vi "Frame to Data.vi"(10 "Frame":string) -> (0 "element":string[](array[string]), 1 "MulFrame":bool, 2 "Array":u8[](array[numeric]), 3 "Get Key？":bool, 4 "Finish":bool, 5 "Error？":bool)   [LabVIEW 2018]
uses:
  <vilib>/regexp/Match Regular Expression.xnode
panel:
  out "Numeric":i32
  out "offset past match":i32
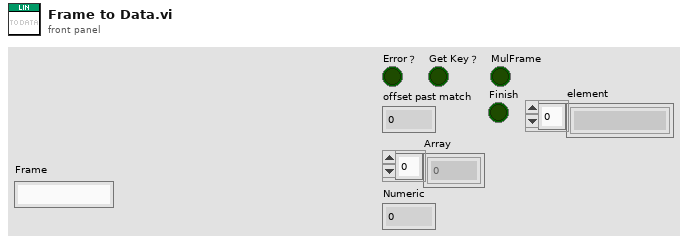
[diagram p1: front panel]
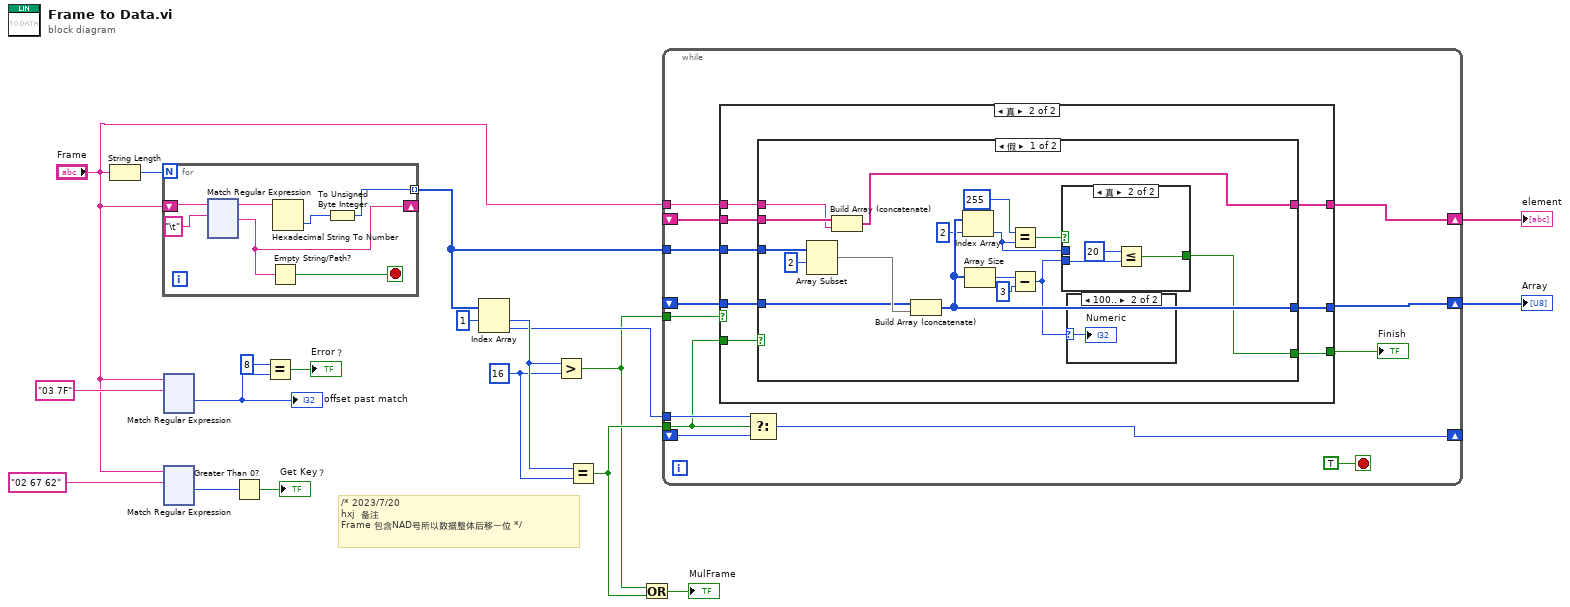
[diagram p0: block diagram]
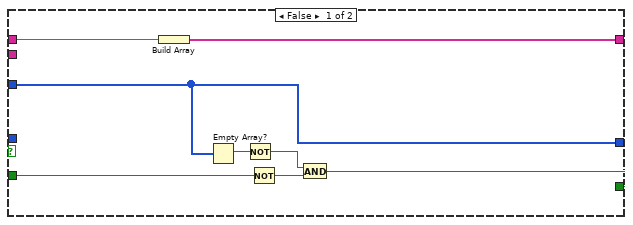
[diagram p2: hidden frame]
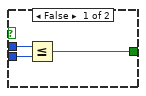
[diagram p4: hidden frame]
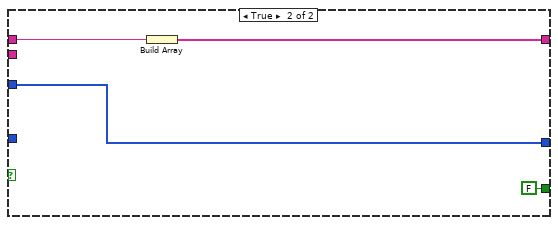
[diagram p5: hidden frame]
diagram:
  w9 = u8 16 ("y")
  # "/* 2023/7/20\nhxj  备注\nFrame 包含NAD号所以数据整体后移一位 */"
  n1 = String Length(string="Frame") -> (length=w19:i32)
  n2 = for {
    N: w19 -> [_]
    shift-right: [w22] -> _
    shift-left: "Frame" -> [w26]
    tunnel: [w23] -> w7 mode=indexing
    stop <- w21 stop-if-true
    n3 = xnode "Match Regular Expression"("input string"=w26, "regular expression"="\t") -> ("before match"=w25:string, "after match"=w22:string)  [unwired: 4 in, 3 out]
    n4 = Empty String/Path?(string/path=w22) -> (empty?=w21:bool)
    n5 = Hexadecimal String To Number(string=w25) -> (number=w24:u32)  [unwired: 2 in, 1 out]
    n6 = To Unsigned Byte Integer(number=w24) -> (unsigned 8bit integer=w23:u8)
  }
  n7 = xnode "Match Regular Expression"("input string"="Frame", "regular expression"="03 7F") -> ("offset past match"=w16:i32)  [unwired: 4 in, 4 out]
  "offset past match" <- w16
  n8 = xnode "Match Regular Expression"("input string"="Frame", "regular expression"="02 67 62") -> ("offset past match"=w13:i32)  [unwired: 4 in, 4 out]
  n9 = Greater Than 0?(x=w13) -> (x > 0?=→"Get Key？":bool)
  n10 = Equal?(x=8, y=w16) -> (x = y?=→"Error？":bool)
  n11 = Index Array(array=w7, index #1=1 ("index")) -> (element #1=w10:u8, element #2=w5:u8)  [unwired: 1 in]
  n12 = Greater?(x=w10, y=w9) -> (0:w4:bool)
  n13 = Equal?(x=w10, y=w9) -> (x = y?=w6:bool)
  n14 = Or(x=w4, y=w6) -> (x .or. y?=→"MulFrame":bool)
  n15 = while {
    tunnel: w7 -> [w145]
    tunnel: w6 -> [w143]
    tunnel: w5 -> [w150]
    shift-right: [w149] -> _
    shift-left: _ -> [w148]
    tunnel: w4 -> [w146]
    tunnel: "Frame" -> [w144]
    shift-right: [w142] -> w2
    shift-left: _ -> [w141]
    shift-right: [w140] -> w1
    shift-left: _ -> [w139]
    stop <- TRUE stop-if-true
    n16 = case shown="真" w146 {
      tunnel: w145 -> [w156 w165]
      tunnel: w144 -> [w158 w162]
      tunnel: w143 -> [w153 w166]
      tunnel: [w156 w164] -> w142
      tunnel: w141 -> [_ w163]
      tunnel: [w157 w161] -> w140
      tunnel: w139 -> [_ w160]
      tunnel: [w151 w159] -> w138
      frame False {
        n17 = Build Array(w158) -> (w157:string[])
        n18 = Empty Array?(array=w156) -> (empty?=w155:bool)
        n19 = Not(x=w155) -> (.not. x?=w154:bool)
        n20 = Not(x=w153) -> (.not. x?=w152:bool)
        n21 = And(x=w154, y=w152) -> (x .and. y?=w151:bool)
      }
      frame True {
        n22 = case shown="假" w166 {
          tunnel: w165 -> [w182 w191]
          tunnel: [w176 w191] -> w164
          tunnel: w163 -> [w179 _]
          tunnel: w162 -> [w170 w193]
          tunnel: [w169 w192] -> w161
          tunnel: w160 -> [w171 _]
          tunnel: [w168 FALSE] -> w159
          frame False {
            n23 = Array Subset(array=w182, index=2) -> (w180:u8[])  [unwired: 1 in]
            n24 = Build Array (concatenate)(w171, w170) -> (w169:string[])
            n25 = Build Array (concatenate)(w179, w180) -> (w176:u8[])
            n26 = Index Array(array=w176, index=2) -> (element=w172:u8)
            n27 = Array Size(array=w176) -> (size(s)=w178:i32)
            n28 = Equal?(x=u8 255 ("y"), y=w172) -> (x = y?=w174:bool)
            n29 = Subtract(x=w178, y=3) -> (x-y=w167:i32)
            n30 = case shown="真" w174 {
              tunnel: w172 -> [w186 _]
              tunnel: w167 -> [w185 w189]
              tunnel: [w184 w187] -> w168
              frame False {
                n31 = Less Or Equal?(x=w186, y=w185) -> (x <= y?=w184:bool)
              }
              frame True {
                n32 = Less Or Equal?(x=20, y=w189) -> (x <= y?=w187:bool)
              }
            }
            n33 = case shown="100.." w167 {
              selector: w167 -> [_ w183]
              frame Default {
              }
              frame 100.. {
                "Numeric" <- w183
              }
            }
          }
          frame True {
            n34 = Build Array(w193) -> (w192:string[])
          }
        }
      }
    }
    "Finish" <- w138
    n35 = Select(t=w150, s=w143, f=w148) -> (s? t:f=w149:u8)
  }
  "Array" <- w2
  "element" <- w1
